vi "Configure Trigger (CAN - Frame).vi"(0 "VISA resource name":refnum<visa-resource-name>, 1 "Data Threshold (0.0V)":dbl, 2 "Nominal Bit Rate (1MB)":dbl=1000000.0, 3 "CAN Format (0:Standard)":u16(ring) items=["Standard", "Extended"], 5 "Source (0:Channel1)":u16(ring) items=["Channel1", "Channel2", "Channel3", "Channel4"], 7 "Signal Type (0:Differential)":u16(ring) items=["Differential", "CAN + H", "CAN - L", "TX", "RX"], 11 "error in (no error)":errorcluster, 12 "Type of Frame (0:Data)":u16(ring) items=["Data", "Remote"]) -> (4 "VISA resource name out":refnum<visa-resource-name>, 15 "error out":errorcluster)   [LabVIEW 2011, in "Tektronix 7000 Series.lvlib"]
doc: "Configures CAN trigger settings (Frame) for an oscilloscope. A trigger occurs when a Controller Area Network frame signal is found.\n\nOnly DPO7000 series oscilloscopes supports CAN triggers."
uses:
  Tektronix 7000 Series.lvlib
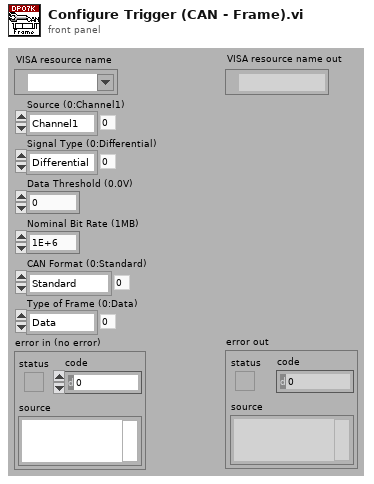
[diagram p1: front panel]
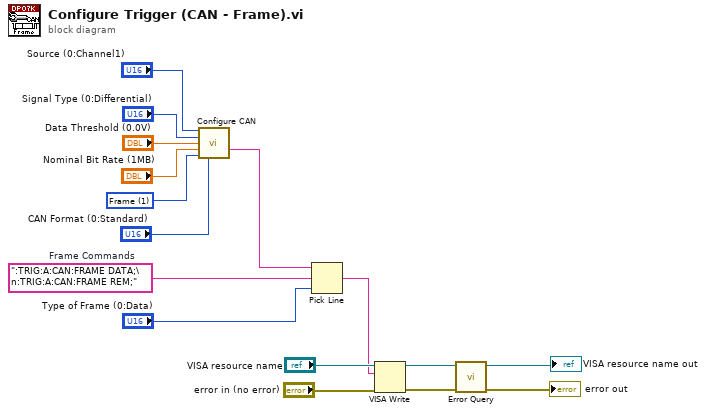
[diagram p0: block diagram]
diagram:
  w8 = ":TRIG:A:CAN:FRAME DATA;\n:TRIG:A:CAN:FRAME REM;"  # Frame Commands
  w12 = u16 1 items=["Start", "Frame", "Identifier", "Data", "Identifier And Data", "EOF", "Missing ack"] ("Trigger Condition (0:Start)")
  n1 = call "Configure CAN.vi"("Source (0:Channel1)"="Source (0:Channel1)", "Signal Type (0:Differential)"="Signal Type (0:Differential)", "Data Threshold (0.0V)"="Data Threshold (0.0V)", "Nominal Bit Rate (1MB)"="Nominal Bit Rate (1MB)", "Trigger Condition (0:Start)"=w12, "CAN Format (0:Standard)"="CAN Format (0:Standard)") -> ("Output String"=w10:string)  [unwired: 9 in]
  n2 = Pick Line(string ("")=w10, multi-line string=w8, line index="Type of Frame (0:Data)") -> (output string=w1:string)
  n3 = VISA Write(VISA resource name="VISA resource name", write buffer=w1, error in (no error)="error in (no error)") -> (VISA resource name out=w7:refnum<visa-resource-name>, error out=w6:errorcluster)  [unwired: 1 out]
  n4 = call "Error Query.vi"("error in (no error)"=w6, "VISA resource name"=w7) -> ("error out"=→"error out":errorcluster, "VISA resource name out"=→"VISA resource name out":refnum<visa-resource-name>)  [unwired: 6 in, 2 out]
